vi "ActorDatabase-UpdateInstructions.vi"(8 "error in (no error)":errorcluster, 11 "Database-Actor in":refnum<class "Database-Actor.lvclass">=refnum) -> (0 "error out":errorcluster, 3 "Database-Actor out":refnum<class "Database-Actor.lvclass">)   [LabVIEW 2013, in "Database-Actor.lvclass"]
uses:
  Database-Actor.lvclass
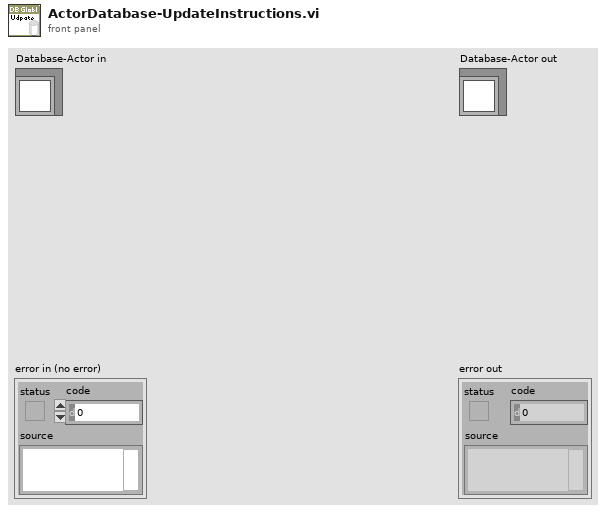
[diagram p1: front panel]
types:
  T1 = cluster{"Table":string, "SQL Statement":string, "Update All":bool, "Payload":string, "Column Number":i32, "Datatype":i32, "Reply Command":string}
  T2 = cluster{"Manufacturing-Part Number":string, string, "Label Instructions":string, "Path for Picture Label":path, "Path for Picture Label 2":path, "Path for Picture Label 3":path, "Path for Picture Label 4":path, "Path for Picture Label 5":path, "Path for Picture Label 6":path, "Path for Picture Label 7":path, "General Instruction Name":string}[]
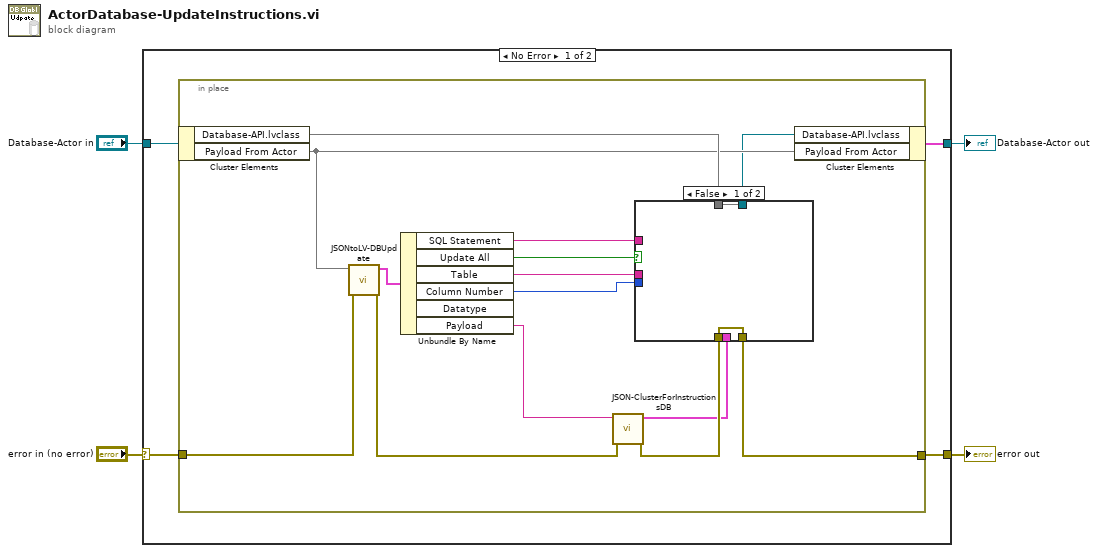
[diagram p0: block diagram]
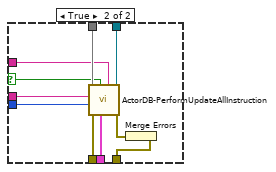
[diagram p2: hidden frame]
diagram:
  n1 = case shown="No Error" "error in (no error)" {
    selector: "error in (no error)" -> [w6 w36]
    tunnel: [w5 w36] -> w3
    tunnel: [w7 w35] -> w1
    tunnel: "Database-Actor in" -> [w8 w35]
    frame No Error {
      n2 = in-place {
        in-place-border: w6 -> [w18]
        in-place-border: [w9] -> w5
        n3 = in-place-cluster #1(w8) -> ("Database-API.lvclass"=w22, "Payload From Actor"=w16)
        n4 = call "JSONtoLV-DBUpdate.vi"("error in"=w18, "Input JSON Object"=w16) -> ("error out"=w14:errorcluster, "value"=w17:T1)  [unwired: 8 in]
        n5 = Unbundle By Name(w17) -> ("SQL Statement"=w21:string, "Update All"=w10:bool, "Table"=w20:string, "Column Number"=w19:i32, "Payload"=w15:string)  [unwired: 1 out]
        n6 = call "JSON-ClusterForInstructionsDB.vi"("error in (no error)"=w14, "Payload"=w15) -> ("error out"=w13:errorcluster, "Cluster Out"=w12:T2)  [unwired: 8 in]
        n7 = case shown="False" w10 {
          selector: w10 -> [_ w27]
          tunnel: w22 -> [w24 w34]
          tunnel: w21 -> [_ w33]
          tunnel: w20 -> [_ w32]
          tunnel: w19 -> [_ w31]
          tunnel: w13 -> [w23 w30]
          tunnel: w12 -> [_ w29]
          tunnel: [w23 w25] -> w9
          tunnel: [w24 w28] -> w11
          frame False {
          }
          frame True {
            n8 = call "ActorDB-PerformUpdateAllInstruction.vi"("SQL Statement"=w33, "Cluster Out"=w29, "Update All"=w27, "error in (no error)"=w30, "Column Number"=w31, "Table"=w32, "Database-API in"=w34) -> ("Error Out"=w26:errorcluster[], "Database-API out"=w28:refnum<class "Database-API.lvclass">)  [unwired: 3 in]
            n9 = Merge Errors(w26) -> (w25:errorcluster)
          }
        }
        n10 = in-place-cluster #1("Database-API.lvclass"=w11, "Payload From Actor"=w16) -> (w7:cluster{})
      }
    }
    frame Error {
    }
  }
  "error out" <- w3
  "Database-Actor out" <- w1
